vi "niDAQmx Create Virtual Channel.vi"   [LabVIEW 2021, in "Session Management niDAQmx.lvlib" / "Session Factory.lvclass"]
doc: "Creates a virtual channel or set of virtual channels and adds them to a task. The instances of this polymorphic VI correspond to the I/O type of the channel, such as analog input, digital output, or counter output; the measurement or generation to perform, such as temperature measurement, voltage generation, or event counting; and in some cases, the sensor to use, such as a thermocouple or RTD for temperature measurements."
uses:
  Session Factory.lvclass
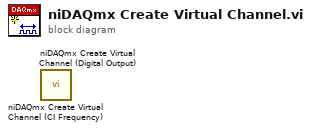
[diagram p0: block diagram]
diagram:
  n1 = call "niDAQmx Create Virtual Channel (CI Frequency).vi"() -> ()  [unwired: 14 in, 2 out]
  n2 = call "niDAQmx Create Virtual Channel (Digital Output).vi"() -> ()  [unwired: 14 in, 2 out]
